vi "Robot Global Data.vi"() -> ()   [LabVIEW 2012]
doc: "This global VI can contain as many global variables as you need. Place a control on the panel, give it a good name. To read or write to it from a VI, drag the icon to the diagram of that VI. You can also drag from the project. Click on the node to change which global you access. You shouldn't have multiple locations writing to a global or it will cause a race-condition."
uses:
  <vilib>/Rock Robotics/WPI/Camera/WPI_CameraImageSize.ctl
  <vilib>/Rock Robotics/WPI/DriverStation/WPI_DriverStationRobotMode2.ctl
  LoopDisable.ctl
panel:
  in  "cResetAngleEncoder":bool
  in  "cQuickShoot":bool
  in  "cDriveAlign":bool
  in  "cFeederAngle":bool
  in  "cReverseDrive":bool
  out "LauncherAngleMatches":bool
  in  "cShield":bool
  in  "sDriveRateL":dbl
  in  "sDriveRateR":dbl
  in  "DisableCluster":T1={"Climb.vi"=TRUE, "LauncherAngle.vi"=TRUE, "Launcher.vi"=TRUE, "ArmControl.vi"=TRUE, "WinchMotor.vi"=TRUE, "ReadDriveEncoder.vi"=FALSE}
  in  "cLauncherAngle":bool
  in  "AutoClimb":bool
  in  "cSolenoidOff":bool
  in  "cHooksIn":bool
  in  "cHooksOut":bool
  in  "sLauncherAngle":dbl
  in  "sLauncherRPM":dbl
  in  "cStraightDrive":bool
  in  "cArmControl":dbl(slide) step=0.2 scale=-1.0..1.0 scale format="%#_3g"
  in  "cClimbReset":bool
  in  "cClimbResume":bool
  in  "cClimbFailSafe":bool
  in  "cClimbStart":bool
  in  "sDriveDistance":dbl
  in  "LauncherTargetAngle":dbl
  in  "LauncherTargetRPM":dbl
  in  "cCalculateFromVision":bool
  in  "cPresetPyramid":bool
  in  "cPresetShort":bool
  in  "cPresetMid":bool
  in  "cPresetFar":bool
  in  "cLauncherWheel":bool
  in  "cFirePneumatic":bool
  in  "cRpmControl":dbl(slide) step=0.2 scale=-1.0..1.0 scale format="%#_3g"
  in  "cAngleControl":dbl(slide) step=0.2 scale=-1.0..1.0 scale format="%#_3g"
  in  "cHalfSpeed":bool
  in  "sGyro":dbl
  in  "ControlOverride":bool
  in  "cTankDriveRight":dbl(slide) step=0.2 scale=-1.0..1.0 scale format="%#_3g"
  in  "cTankDriveLeft":dbl(slide) step=0.2 scale=-1.0..1.0 scale format="%#_3g"
  in  "Robot Mode":T2
  in  "LED toggle rate (ms)":u32=20
  in  "image size":T3=enum."320x240"
  in  "Enable Vision":bool
  # "DRIVER"
  # "SHOOTER"
  # "TODO: Climbing controls for driver"
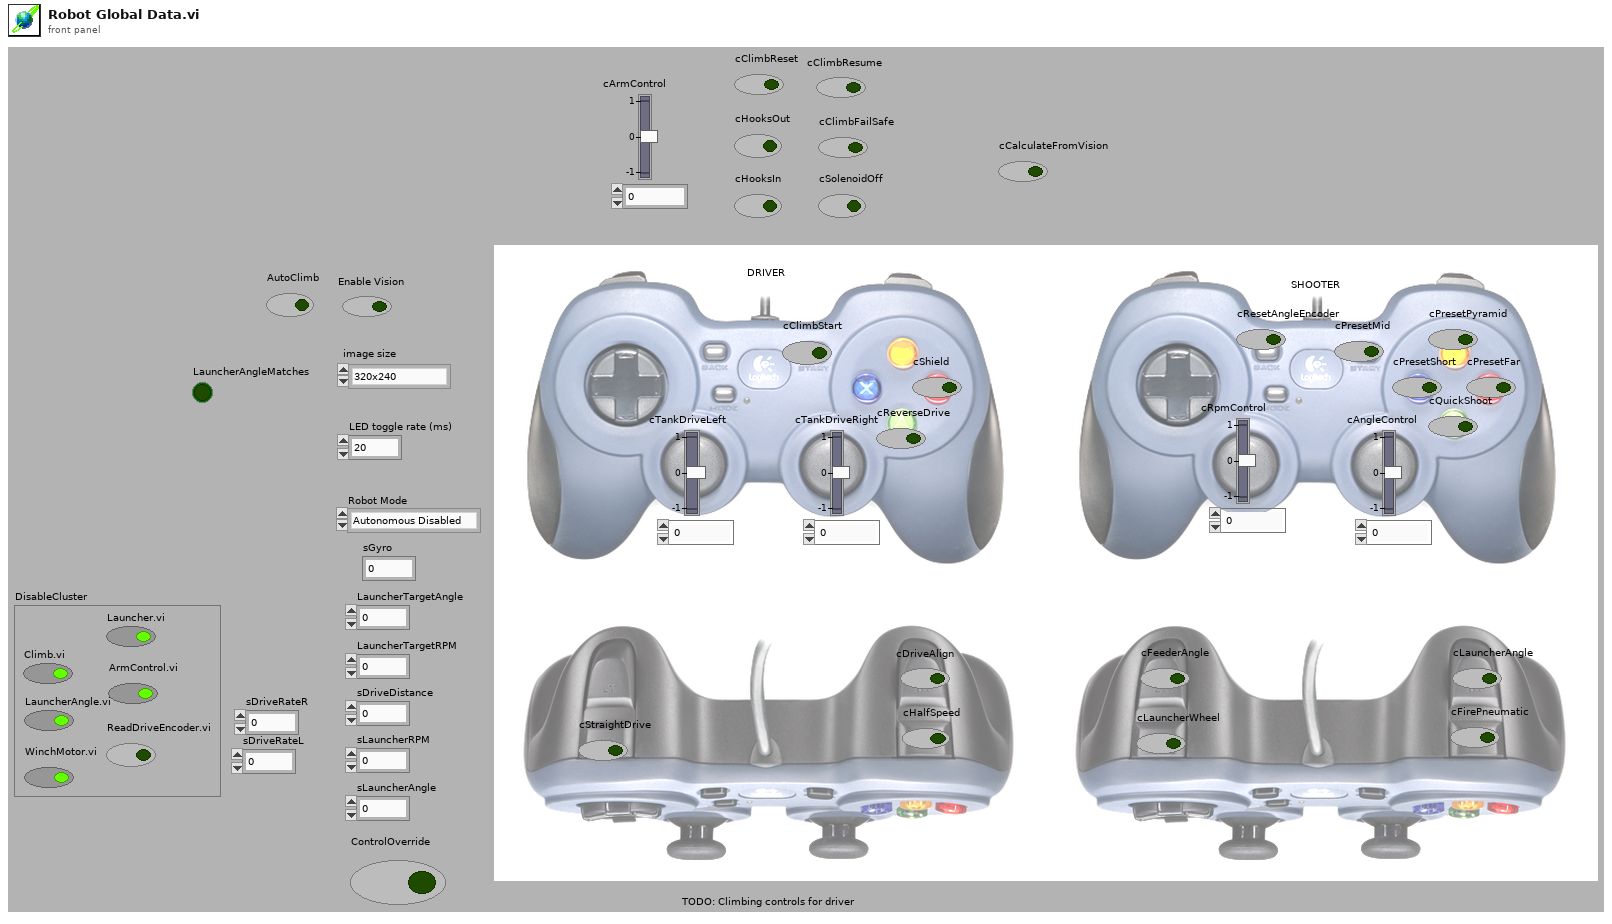
[diagram p1: front panel]
types:
  T1 = typedef "LoopDisable.ctl" = cluster{"Climb.vi":bool, "LauncherAngle.vi":bool, "Launcher.vi":bool, "ArmControl.vi":bool, "WinchMotor.vi":bool, "ReadDriveEncoder.vi":bool}
  T2 = typedef "WPI_DriverStationRobotMode2.ctl" = enum16{"Autonomous Disabled", "Autonomous Enabled", "Teleop Disabled", "Teleop Enabled", "Timeout", "Finish", "Test Disabled", "Test Enabled"}
  T3 = typedef "WPI_CameraImageSize.ctl" = enum16{"640x480", "320x240", "160x120"}
diagram:
